vi "getSymboleResampled.vi"(8 "error in (no error)":errorcluster, 10 "Multiplier":dbl=4.0, 11 "Waveform":waveform(dbl)) -> (0 "error out":errorcluster, 3 "resampled waveform out":waveform(dbl))   [LabVIEW 2018]
uses:
  <vilib>/measure/maresamp.llb/Resample Waveform (single shot).vi
  <vilib>/measure/NI_MAPro.lvlib
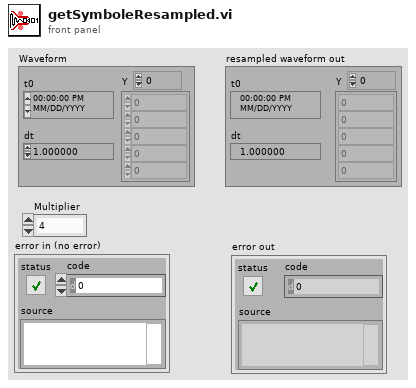
[diagram p1: front panel]
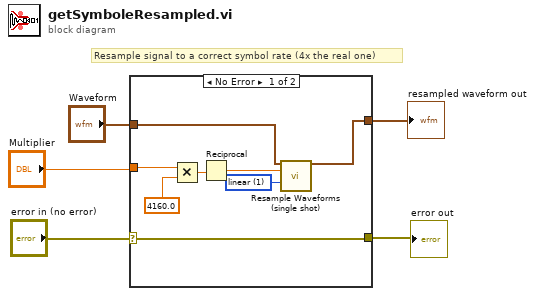
[diagram p0: block diagram]
diagram:
  # "Resample signal to a correct symbol rate (4x the real one)"
  n1 = case shown="No Error" "error in (no error)" {
    selector: "error in (no error)" -> [w9 w14]
    tunnel: [w13 w15] -> w5
    tunnel: "Waveform" -> [w10 w15]
    tunnel: [w9 w14] -> w2
    tunnel: "Multiplier" -> [w6 _]
    frame No Error {
      w12 = u16 1 items=["coerce", "linear", "spline", "FIR filter"] ("interpolation mode")
      n2 = Multiply(x=w6, y=4160.0) -> (x*y=w8:dbl)
      n3 = Reciprocal(x=w8) -> (1/x=w11:dbl)
      n4 = call-poly <vilib>:"Resample Waveforms (single shot).vi"("waveform in"=w10, "dt"=w11, "interpolation mode"=w12) -> ("resampled waveform out"=w13:waveform(dbl))  [unwired: 9 in, 3 out]
    }
    frame Error {
    }
  }
  "resampled waveform out" <- w5
  "error out" <- w2
